vi "FileWriteTest.vi"() -> ()   [LabVIEW 2017]
panel:
  in  "stop":bool
  out "Error Out":errorcluster
  in  "FileFormat":string[](array[string])=["%.1f", "%d", "%.6f"]
  in  "Labels":string[](array[string])=["Ones", "Twos", "Threes"]
  in  "file path (use dialog)":path=path "C:/LabVIEW/DATA/TestData/test.csv"
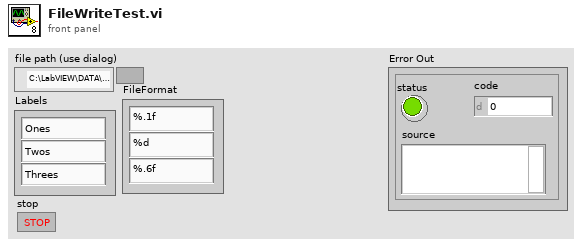
[diagram p1: front panel]
types:
  T1 = enum16{"open", "replace", "create", "open or create", "replace or create", "replace or create with confirmation"}
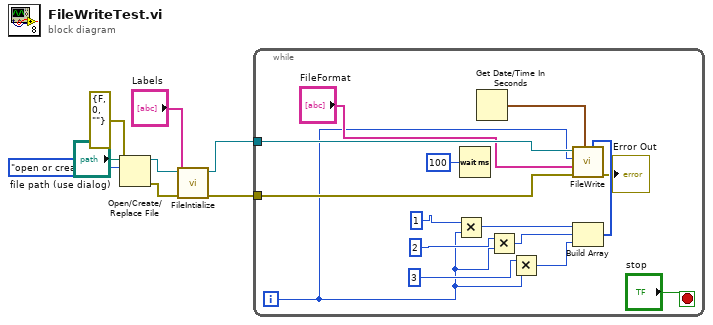
[diagram p0: block diagram]
diagram:
  n1 = Open/Create/Replace File(file path (use dialog)="file path (use dialog)", error in=errorcluster {"status"=FALSE, "code"=0, "source"=""}, operation (0:open)=T1."open or create") -> (refnum out=w7:refnum<file>, error out=w5:errorcluster)  [unwired: 3 in, 1 out]
  n2 = call "FileIntialize.vi"("Error In"=w5, "Labels"="Labels", "refnum in"=w7) -> ("Error Out"=w2:errorcluster, "File Refnum"=w3:refnum<file>)  [unwired: 7 in]
  n3 = while {
    tunnel: w3 -> [w14]
    tunnel: w2 -> [w13]
    i -> [w11]
    stop <- "stop" stop-if-true
    n4 = Multiply(x=1, y=w11) -> (x*y=w19:i32)
    n5 = Wait (ms)(milliseconds to wait=u32 100) -> ()  [unwired: 1 out]
    n6 = Get Date/Time In Seconds() -> (seconds since 1Jan1904=w16:timestamp)
    n7 = Multiply(x=2, y=w11) -> (x*y=w18:i32)
    n8 = Multiply(x=3, y=w11) -> (x*y=w17:i32)
    n9 = Build Array(w19, w18, w17) -> (w15:i32[])
    n10 = call "FileWrite.vi"("DataArray"=w15, "Time Stamp"=w16, "Error In"=w13, "FileFormat"="FileFormat", "Index"=w11, "refnum in"=w14) -> ("Error Out"=→"Error Out":errorcluster)  [unwired: 4 in, 1 out]
  }
